vi "Time Functions.vi"() -> ()   [LabVIEW 2022 SP3]
panel:
  out "current time":timestamp
  out "time string":string
  out "date string":string
  in  "date format (0)":enum16{"short", "long", "abbreviated"}(ring)
  out "x+y":i32
  out "millisecond timer value 3":u32
  out "millisecond timer value 2":u32
  out "relative seconds":dbl format="%_19f"
  out "millisecond timer value":u32
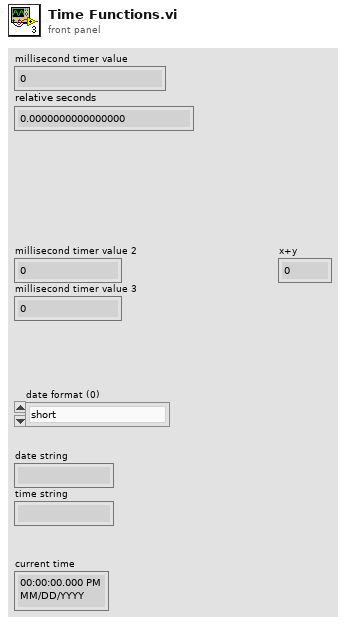
[diagram p1: front panel]
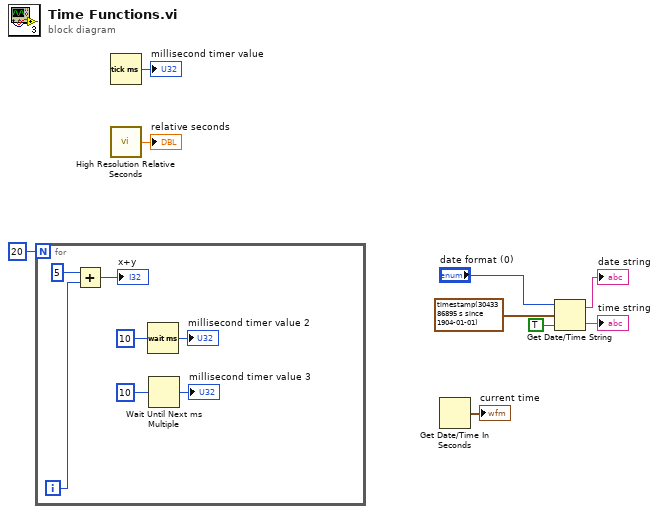
[diagram p0: block diagram]
diagram:
  n1 = for {
    N: 20 -> [_]
    i -> [w12]
    n2 = Add(x=5, y=w12) -> (x+y=→"x+y":i32)
    n3 = Wait (ms)(milliseconds to wait=u32 10 ("millisecond timer value")) -> (millisecond timer value=→"millisecond timer value 2":u32)
    n4 = Wait Until Next ms Multiple(millisecond multiple=u32 10 ("millisecond timer value")) -> (millisecond timer value=→"millisecond timer value 3":u32)
  }
  n5 = Tick Count (ms)() -> (millisecond timer value=→"millisecond timer value":u32)
  n6 = call <vilib>:"High Resolution Relative Seconds.vi"() -> ("relative seconds"=→"relative seconds":dbl)
  n7 = Get Date/Time In Seconds() -> (seconds since 1Jan1904=→"current time":timestamp)
  n8 = Get Date/Time String(date format (0)="date format (0)", seconds (now)=timestamp(3043386895 s since 1904-01-01), want seconds? (F)=TRUE) -> (date string=→"date string":string, time string=→"time string":string)
